vi "TestMulticolumnListboxAccess.vi"(8 "error in (no error)":errorcluster) -> (0 "error out":errorcluster)   [LabVIEW 2016, in "WeatherReportTests.lvlib"]
uses:
  WeatherReportTests.lvlib
  APIs/Stimulus/ControlValue/Controls/MC Listbox/SetValueByItemName.vi
  APIs/Assert/AssertControlValue/Equal.vi
  APIs/Stimulus/VI/CloseVI.vi
  <vilib>/addons/_JKI Toolkits/Caraya/classes/Test/Test.lvclass
  Drona.lvlib
  APIs/Assert/AssertControlValue/AssertControlValue.lvlib
  APIs/Stimulus/VI/VI.lvlib
  APIs/Stimulus/ControlValue/Controls/MC Listbox/StimulusMCListbox.lvlib
panel:
  # "Drona Test Multicolumn Access"
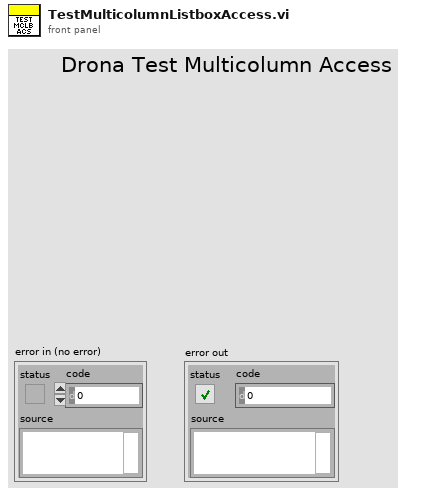
[diagram p1: front panel]
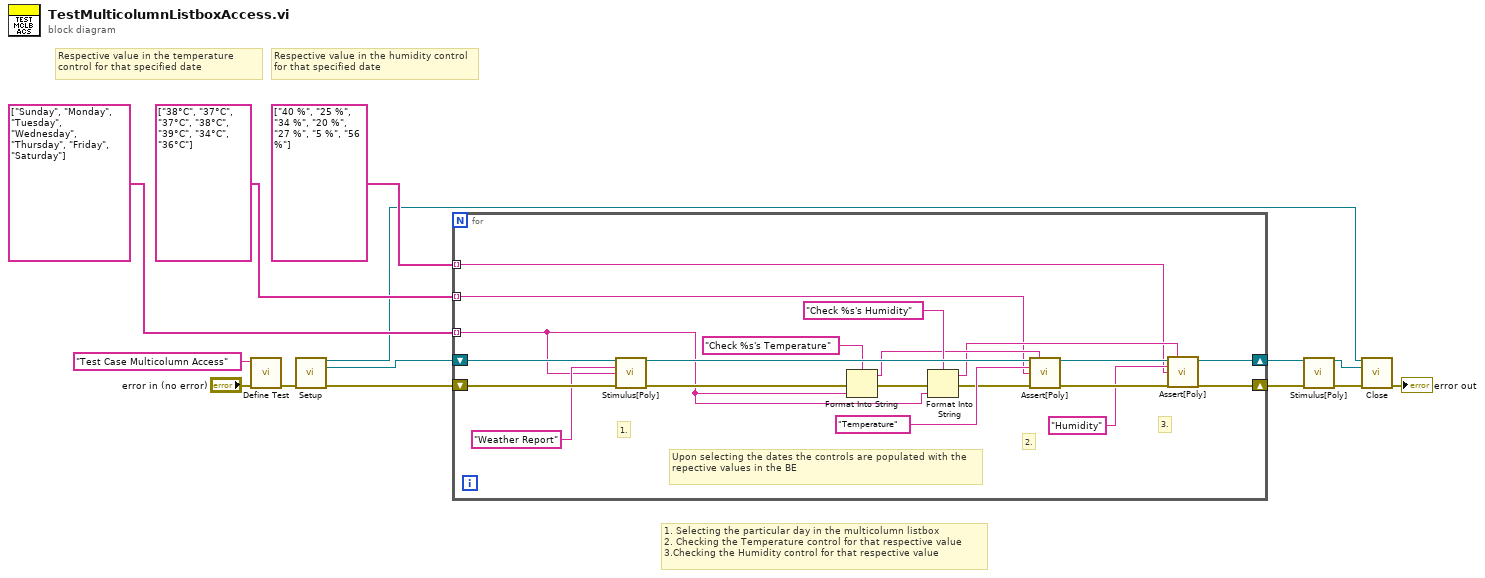
[diagram p0: block diagram]
diagram:
  # "1. Selecting the particular day in the multicolumn listbox\n2. Checking the Temperature control for that respective value\n3.Checking the Humidity control for that respective value"
  # "Respective value in the humidity control for that specified date"
  # "Respective value in the temperature control for that specified date"
  n1 = call <vilib>:"Define Test.vi"("error in (no error)"="error in (no error)", "Label (VI Title)"="Test Case Multicolumn Access") -> ("error out"=w12:errorcluster)  [unwired: 8 in, 1 out]
  n2 = call "Setup.vi"("error in"=w12) -> ("Application Ref"=w1:refnum<vi>, "VI Reference Out"=w11:refnum<vi>, "error out"=w10:errorcluster)  [unwired: 12 in]
  n3 = for {
    shift-right: [w28] -> w5
    shift-left: w11 -> [w34]
    shift-right: [w29] -> w6
    shift-left: w10 -> [w33]
    tunnel: string[] ["Sunday", "Monday", "Tuesday", "Wednesday", "Thursday", "Friday", "Saturday"] ("Item Name") -> [w17] mode=indexing
    tunnel: string[] ["38°C", "37°C", "37°C", "38°C", "39°C", "34°C", "36°C"] ("Control Path") -> [w15] mode=indexing
    tunnel: string[] ["40 %", "25 %", "34 %", "20 %", "27 %", "5 %", "56 %"] ("Control Path") -> [w16] mode=indexing
    # "Upon selecting the dates the controls are populated with the repective values in the BE"
    # "3."
    # "2."
    # "1."
    n4 = call-poly "Stimulus[Poly].vi"("VI Reference In"=w34, "Control Path"="Weather Report", "Item Name"=w17, "Error In"=w33) -> ("VI Reference Out"=w31:refnum<vi>, "Error Out"=w30:errorcluster)  [unwired: 10 in]
    n5 = Format Into String(format string="Check %s's Temperature", error in=w30, w17) -> (resulting string=w19:string, error out=w21:errorcluster)  [unwired: 1 in]
    n6 = Format Into String(format string="Check %s's Humidity", error in=w21, w17) -> (resulting string=w18:string, error out=w20:errorcluster)  [unwired: 1 in]
    n7 = call-poly "Assert[Poly].vi"("VI Reference In"=w31, "Test Label"=w19, "Control Path"="Temperature", "Control Value"=w15, "Error In"=w20) -> ("VI Reference Out"=w25:refnum<vi>, "Error Out"=w26:errorcluster)  [unwired: 8 in, 1 out]
    n8 = call-poly "Assert[Poly].vi"("VI Reference In"=w25, "Test Label"=w18, "Control Path"="Humidity", "Control Value"=w16, "Error In"=w26) -> ("VI Reference Out"=w28:refnum<vi>, "Error Out"=w29:errorcluster)  [unwired: 8 in, 1 out]
  }
  n9 = call-poly "Stimulus[Poly].vi"("VI Reference In"=w5, "error in"=w6) -> ("VI Reference Out"=w7:refnum<vi>, "error out"=w8:errorcluster)  [unwired: 12 in]
  n10 = call "Close.vi"("Application Ref"=w1, "VI Reference"=w7, "error in"=w8) -> ("error out"=→"error out":errorcluster)  [unwired: 12 in]
